vi "Open Device (serial number).vi"(8 "error in (no error)":errorcluster, 10 "Device Serial Number":string) -> (0 "error out":errorcluster, 3 "Handle":u64)   [LabVIEW 2019, in "D2XX-lv.lvlib"]
doc: "Open the specified device and return a handle that will be used for subsequent accesses. The device is specified by its serial number."
uses:
  D2XX-lv.lvlib
  <instrlib>/_D2XX/D2XX/D2XX.lvlib
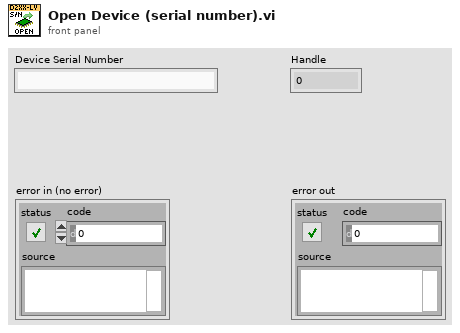
[diagram p1: front panel]
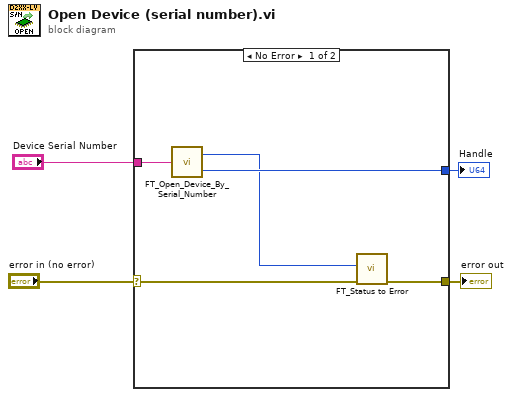
[diagram p0: block diagram]
diagram:
  n1 = case shown="No Error" "error in (no error)" {
    selector: "error in (no error)" -> [w9 w10]
    tunnel: [w8 w10] -> w3
    tunnel: "Device Serial Number" -> [w7 _]
    tunnel: [w6 _] -> w1
    frame No Error {
      n2 = call <instrlib>:"FT_Open_Device_By_Serial_Number.vi"("Device Serial Number"=w7) -> ("FT_Status"=w5:u32, "Handle"=w6:u64)
      n3 = call "FT_Status to Error.vi"("error in (no error)"=w9, "FT_Status"=w5) -> ("error out"=w8:errorcluster)  [unwired: 9 in]
    }
    frame Error {
    }
  }
  "error out" <- w3
  "Handle" <- w1
